vi "Get Message From Mediator.vi"(8 "error in (no error)":errorcluster caption="错误输入（无错误）", 11 "Mediator 输入":refnum<class "Mediator.lvclass"> caption="DNL_LabVIEW Object in") -> (0 "error out":errorcluster caption="错误输出", 3 "Mediator 输出":refnum<class "Mediator.lvclass"> caption="DNL_LabVIEW Object out")   [LabVIEW 2011, in "Mediator.lvclass"]
uses:
  Mediator.lvclass
  Mediator.lvclass/Mediator.ctl
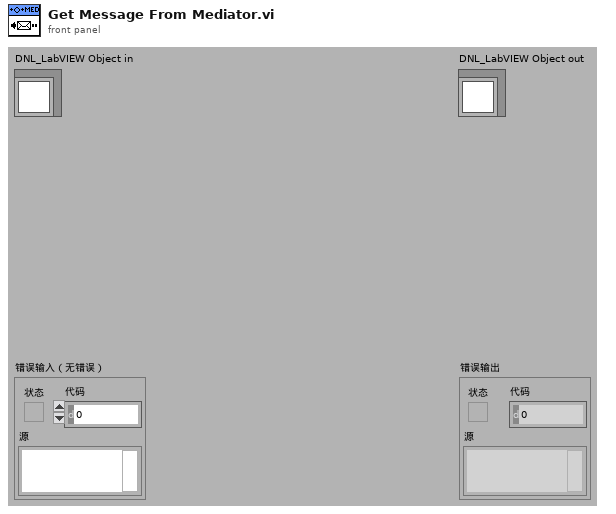
[diagram p1: front panel]
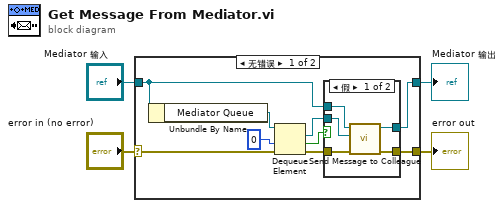
[diagram p0: block diagram]
diagram:
  n1 = case shown="无错误" "error in (no error)" {
    selector: "error in (no error)" -> [w11 w22]
    tunnel: [w5 w22] -> w3
    tunnel: [w7 w21] -> w1
    tunnel: "Mediator 输入" -> [w9 w21]
    frame No Error {
      n2 = Unbundle By Name(w9) -> ("Mediator Queue"=w13:refnum<queue>)
      n3 = Dequeue Element(queue=w13, timeout in ms (-1)=0 ("超时毫秒(-1)"), error in (no error)=w11) -> (element=w8:refnum<class "Message.lvclass">, timed out?=w10:bool, error out=w6:errorcluster)  [unwired: 1 out]
      n4 = case shown="假" w10 {
        tunnel: w9 -> [w18 w20]
        tunnel: w8 -> [w17 _]
        tunnel: [w16 w20] -> w7
        tunnel: w6 -> [w15 w19]
        tunnel: [w14 w19] -> w5
        frame False {
          n5 = call "Send Message to Colleague.vi"("error in (no error)"=w15, "Message.lvclass"=w17, "中介者（抽象） 输入"=w18) -> ("error out"=w14:errorcluster, "中介者（抽象） 输出"=w16:refnum<class "Mediator.lvclass">)  [unwired: 7 in]
        }
        frame True {
        }
      }
    }
    frame Error {
    }
  }
  "error out" <- w3
  "Mediator 输出" <- w1
